vi "StringList.Init.vi"(6 "Bottom Items":string[](array[string]), 7 "Ring Ctrl":refnum<vi>, 8 "error in (no error)":errorcluster, 9 "Default Items":string[](array[string]), 10 "Top Items":string[](array[string]), 11 "StringList in":refnum<class "StringList.lvclass">) -> (0 "error out":errorcluster, 2 "Items Out":string[](array[string]), 3 "StringList out":refnum<class "StringList.lvclass">)   [LabVIEW 2024, in "StringList.lvclass"]
uses:
  StringList.lvclass
  StringList.lvclass/StringList.ctl
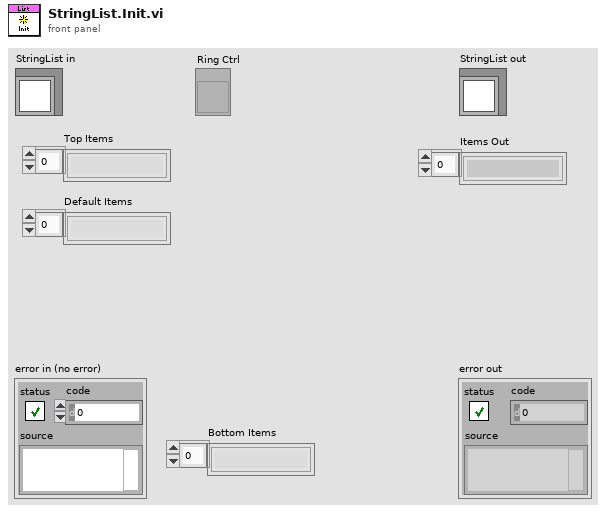
[diagram p1: front panel]
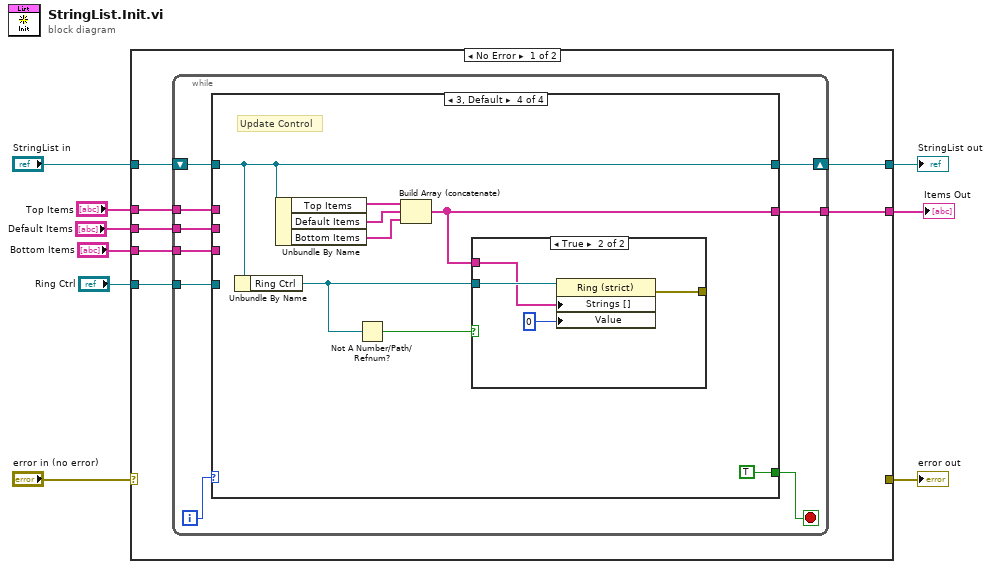
[diagram p0: block diagram]
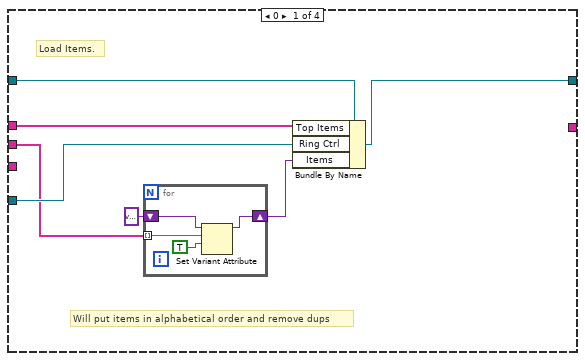
[diagram p2: hidden frame]
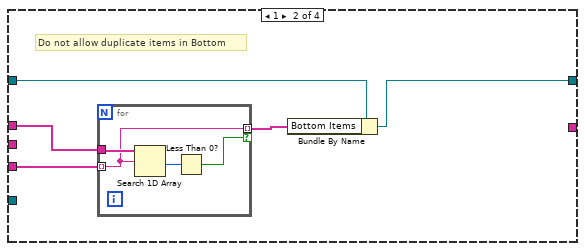
[diagram p3: hidden frame]
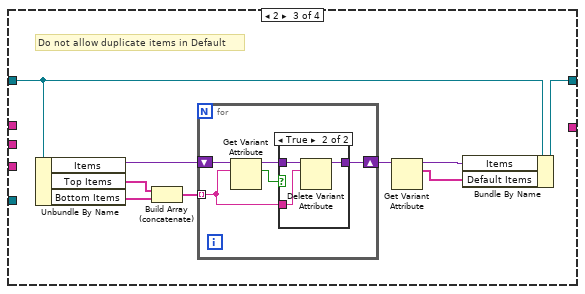
[diagram p4: hidden frame]
diagram:
  n1 = case shown="No Error" "error in (no error)" {
    selector: "error in (no error)" -> [_ w77]
    tunnel: [_ w77] -> w8
    tunnel: [w14 w76] -> w6
    tunnel: "StringList in" -> [w13 w76]
    tunnel: "Top Items" -> [w16 _]
    tunnel: "Ring Ctrl" -> [w12 _]
    tunnel: "Default Items" -> [w11 _]
    tunnel: "Bottom Items" -> [w15 _]
    tunnel: [w10 _] -> w1
    frame No Error {
      n2 = while {
        tunnel: w16 -> [w25]
        tunnel: w15 -> [w24]
        tunnel: w12 -> [w21]
        tunnel: w11 -> [w20]
        shift-right: [w23] -> w14
        shift-left: w13 -> [w22]
        tunnel: [w17] -> w10
        i -> [w19]
        stop <- w18 stop-if-true
        n3 = case shown="3, Default" w19 {
          tunnel: w25 -> [w32 w40 _ _]
          tunnel: w24 -> [_ w41 _ _]
          tunnel: [w31 w38 w54 w71] -> w23
          tunnel: w22 -> [w30 w37 w53 w71]
          tunnel: w21 -> [w29 _ _ _]
          tunnel: w20 -> [w27 _ _ _]
          tunnel: [_ _ _ TRUE] -> w18
          tunnel: [_ _ _ w65] -> w17
          frame 0 {
            # "Will put items in alphabetical order and remove dups"
            # "Load Items."
            n4 = for {
              tunnel: w27 -> [w36] mode=indexing
              shift-right: [w33] -> w26
              shift-left: variant -> [w34]
              n5 = Set Variant Attribute(Variant=w34, name=w36, value=TRUE) -> (Variant out=w33:variant)  [unwired: 1 in, 2 out]
            }
            n6 = Bundle By Name(cluster=w30, "Top Items"=w32, "Ring Ctrl"=w29, "Items"=w26) -> (w31:refnum<class "StringList.lvclass">)
          }
          frame 1 {
            # "Do not allow duplicate items in Bottom"
            n7 = for {
              tunnel: w41 -> [w43] mode=indexing
              tunnel: w40 -> [w45]
              tunnel: [w43] -> w39 mode=indexing if=w42
              n8 = Search 1D Array(1D array=w45, element=w43) -> (index of element=w44:i32)  [unwired: 1 in]
              n9 = Less Than 0?(x=w44) -> (x < 0?=w42:bool)
            }
            n10 = Bundle By Name(cluster=w37, "Bottom Items"=w39) -> (w38:refnum<class "StringList.lvclass">)
          }
          frame 2 {
            # "Do not allow duplicate items in Default"
            n11 = Unbundle By Name(w53) -> ("Items"=w50:variant, "Top Items"=w49:string[], "Bottom Items"=w52:string[])
            n12 = Build Array (concatenate)(w49, w52) -> (w51:string[])
            n13 = for {
              tunnel: w51 -> [w56] mode=indexing
              shift-right: [w55] -> w48
              shift-left: w50 -> [w59]
              n14 = Get Variant Attribute(Variant=w59, name=w56) -> (duplicate Variant=w57:variant, found=w58:bool)  [unwired: 2 in, 2 out]
              n15 = case shown="True" w58 {
                tunnel: w57 -> [w60 w63]
                tunnel: w56 -> [_ w62]
                tunnel: [w60 w61] -> w55
                frame False {
                }
                frame True {
                  n16 = Delete Variant Attribute(6:w62, 7:w63) -> (3:w61:variant)  [unwired: 1 in, 2 out]
                }
              }
            }
            n17 = Get Variant Attribute(Variant=w48) -> (duplicate Variant=w47:variant, names=w46:string[])  [unwired: 3 in, 2 out]
            n18 = Bundle By Name(cluster=w53, "Items"=w47, "Default Items"=w46) -> (w54:refnum<class "StringList.lvclass">)
          }
          frame 3, Default {
            # "Update Control"
            n19 = Unbundle By Name(w71) -> ("Ring Ctrl"=w70:refnum<vi>)
            n20 = Unbundle By Name(w71) -> ("Top Items"=w68:string[], "Default Items"=w67:string[], "Bottom Items"=w66:string[])
            n21 = Not A Number/Path/Refnum?(number/path/refnum=w70) -> (NaN/Path/Refnum?=w64:bool)
            n22 = Build Array (concatenate)(w68, w67, w66) -> (w65:string[])
            n23 = case shown="True" w64 {
              tunnel: w70 -> [_ w75]
              tunnel: w65 -> [_ w73]
              tunnel: [_ w72] -> _
              frame False {
              }
              frame True {
                n24 = property class="Ring (strict)"(reference=w75, "Strings []"=w73, "Value"=u16 0) -> (error out=w72:errorcluster)  [unwired: 1 in, 1 out]
              }
            }
          }
        }
      }
    }
    frame Error {
    }
  }
  "error out" <- w8
  "StringList out" <- w6
  "Items Out" <- w1
